vi "SW_Mix_TTL_inputs.vi"(1 "TTL input 2":u8, 2 "TTL input 1":u8) -> (0 "TTL mixed output":u8)   [LabVIEW 2016]
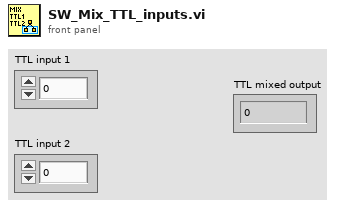
[diagram p1: front panel]
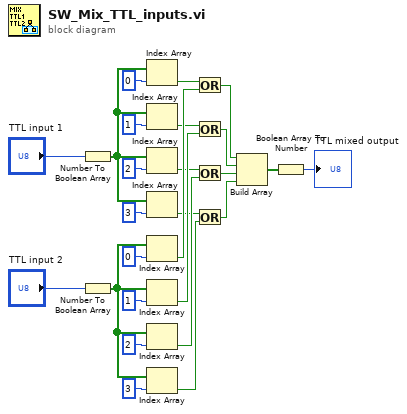
[diagram p0: block diagram]
diagram:
  n1 = Number To Boolean Array(number="TTL input 1") -> (Boolean array=w15:bool[])
  n2 = Number To Boolean Array(number="TTL input 2") -> (Boolean array=w16:bool[])
  n3 = Index Array(array=w15, index=0) -> (element=w14:bool)
  n4 = Index Array(array=w15, index=1) -> (element=w12:bool)
  n5 = Index Array(array=w15, index=2) -> (element=w10:bool)
  n6 = Index Array(array=w15, index=3) -> (element=w8:bool)
  n7 = Index Array(array=w16, index=0) -> (element=w13:bool)
  n8 = Index Array(array=w16, index=1) -> (element=w11:bool)
  n9 = Index Array(array=w16, index=2) -> (element=w9:bool)
  n10 = Index Array(array=w16, index=3) -> (element=w7:bool)
  n11 = Or(x=w14, y=w13) -> (x .or. y?=w6:bool)
  n12 = Or(x=w12, y=w11) -> (x .or. y?=w5:bool)
  n13 = Or(x=w10, y=w9) -> (x .or. y?=w4:bool)
  n14 = Or(x=w8, y=w7) -> (x .or. y?=w3:bool)
  n15 = Build Array(w6, w5, w4, w3) -> (w2:bool[])
  n16 = Boolean Array To Number(Boolean array=w2) -> (number=→"TTL mixed output":u32)
